vi "Multiple QCM VI.vi"() -> ()   [LabVIEW 2014]
uses:
  <vilib>/Utility/error.llb/DialogType.ctl
  <vilib>/Instr/_visa.llb/VISA Configure Serial Port (Instr).vi
  <vilib>/DAQmx/create/channels.llb/DAQmx Create Channel (DO-Digital Output).vi
  <vilib>/DAQmx/write.llb/DAQmx Write (Digital 1D Bool 1Chan 1Samp).vi
  <vilib>/Utility/file.llb/Write To Spreadsheet File (string).vi
  <vilib>/Utility/file.llb/Write To Spreadsheet File (DBL).vi
panel:
  out "x-y 3":dbl
  out "x-y 2":dbl
  out "Numeric":i32
  out "s? t:f 3":dbl
  out "Waveform Chart 8":dbl[](graph) caption="Waveform Chart"
  out "Frequency 3":dbl
  out "X":dbl
  out "x-y":dbl
  out "s? t:f 2":dbl
  out "Waveform Chart 7":dbl[](graph) caption="Waveform Chart"
  out "Y":dbl
  out "Waveform Chart 6":dbl[](graph) caption="Waveform Chart"
  out "y":dbl
  in  "stop":bool
  out "Frequency 2":dbl
  out "Frequency":dbl
  out "Waveform Chart 2":dbl[](graph) caption="Waveform Chart"
  out "Temperature":dbl
  out "Current Channel\nEnabled":dbl
  out "read buffer":string
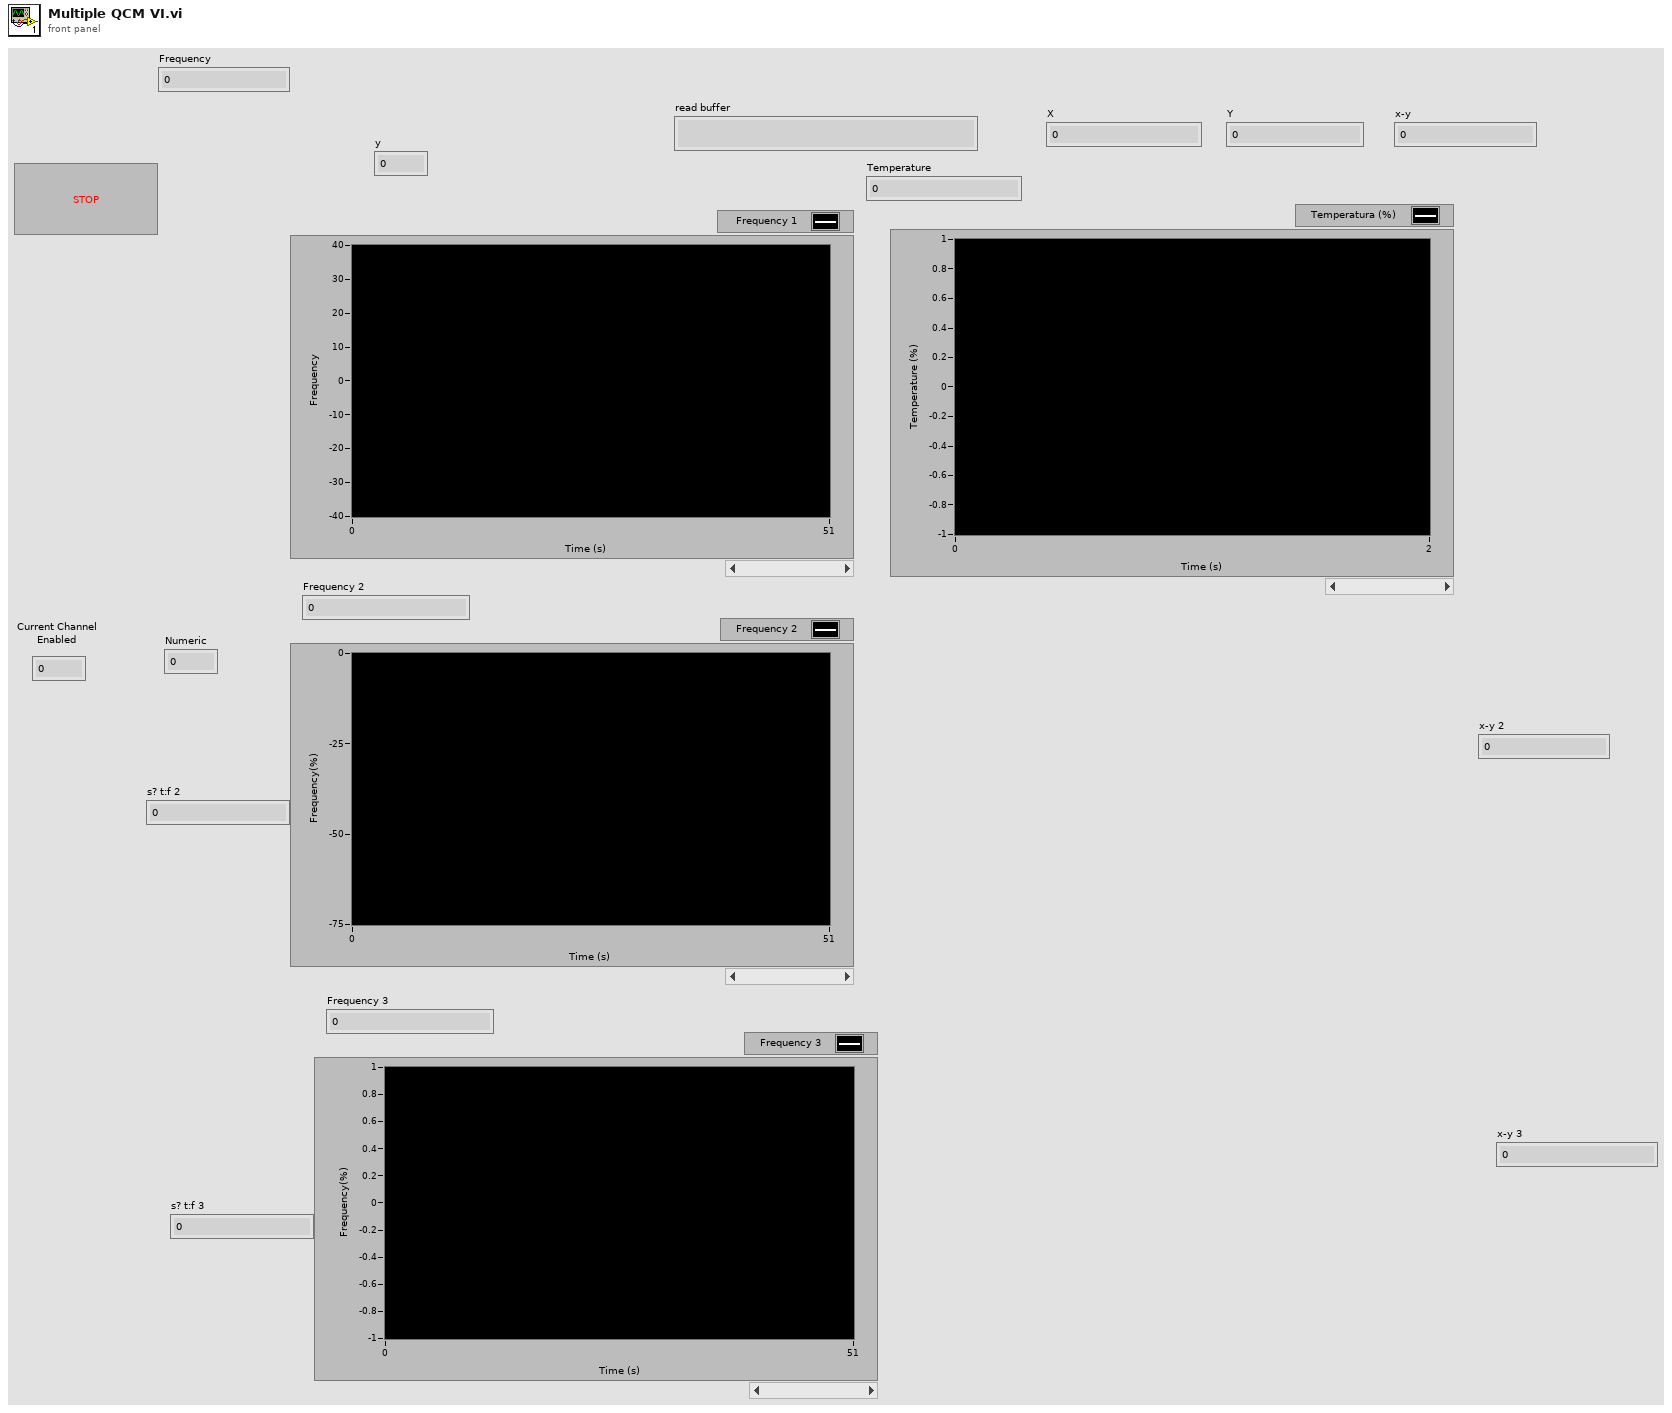
[diagram p1: front panel]
types:
  T1 = typedef "DialogType.ctl" = u16
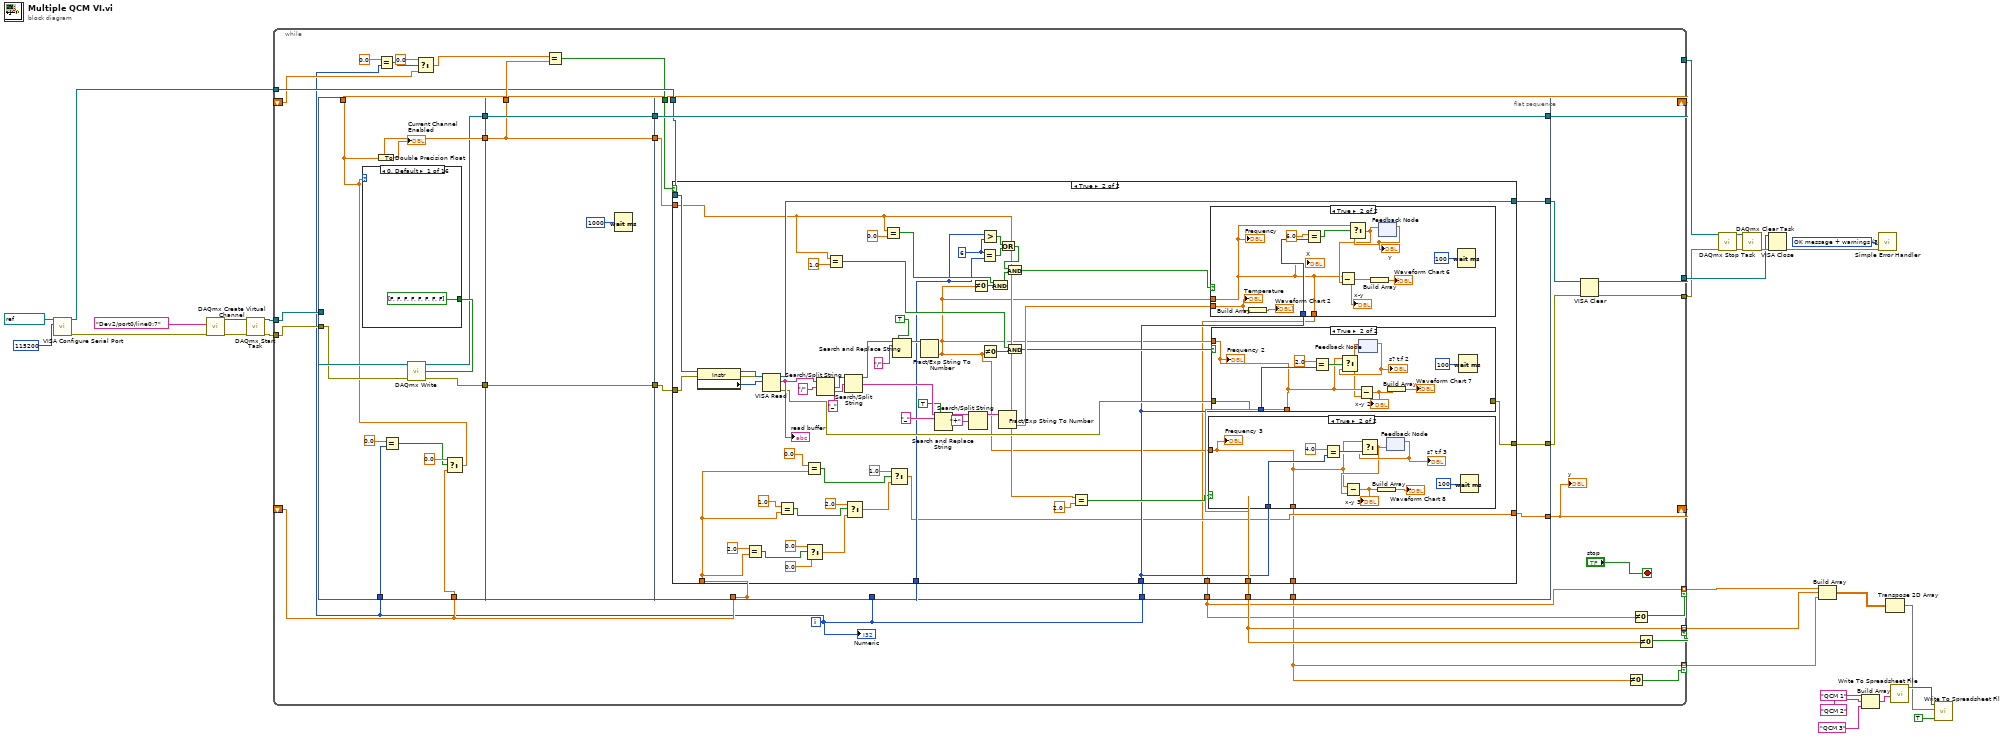
[diagram p0: block diagram]
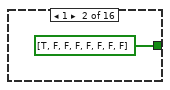
[diagram p2: hidden frame]
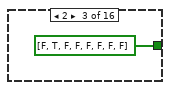
[diagram p3: hidden frame]
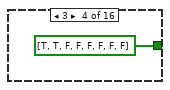
[diagram p4: hidden frame]
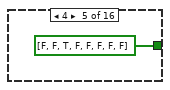
[diagram p5: hidden frame]
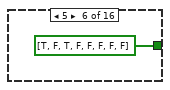
[diagram p6: hidden frame]
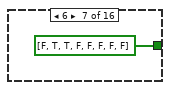
[diagram p7: hidden frame]
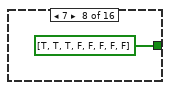
[diagram p8: hidden frame]
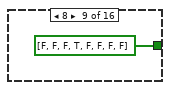
[diagram p9: hidden frame]
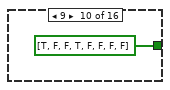
[diagram p10: hidden frame]
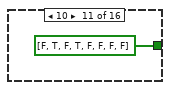
[diagram p11: hidden frame]
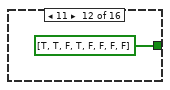
[diagram p12: hidden frame]
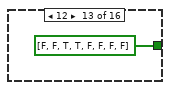
[diagram p13: hidden frame]
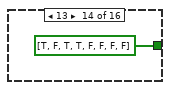
[diagram p14: hidden frame]
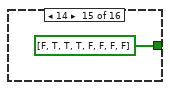
[diagram p15: hidden frame]
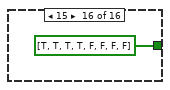
[diagram p16: hidden frame]
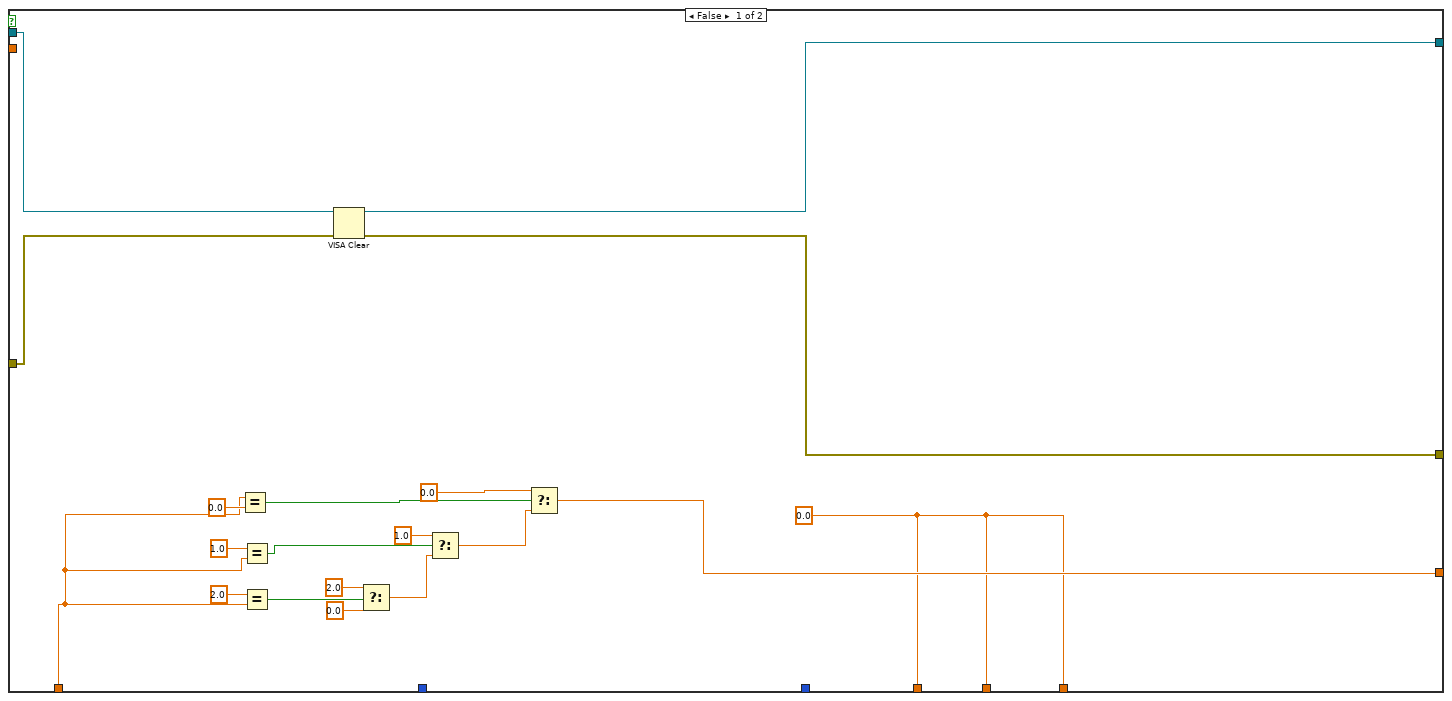
[diagram p17: hidden frame]
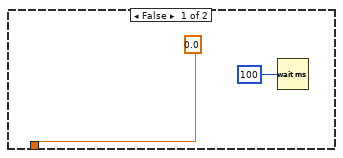
[diagram p18: hidden frame]
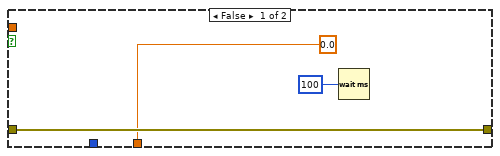
[diagram p19: hidden frame]
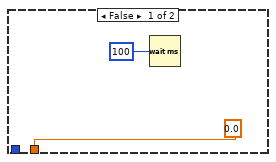
[diagram p20: hidden frame]
diagram:
  w25 = T1 3 items=["no dialog", "OK message", "continue or stop message", "OK message + warnings", "continue/stop + warnings"] ("type of dialog (OK msg:1)")
  n1 = call-poly "VISA Configure Serial Port"("VISA resource name"=refnum<visa-resource-name> "COM12", "baud rate (9600)"=u32 115200) -> ("VISA resource name out"=w28:refnum<visa-resource-name>, "error out"=w19:errorcluster)  [unwired: 12 in]
  n2 = call-poly <vilib>:"DAQmx Create Virtual Channel.vi"("lines"=tag "Dev2/port0/line0:7" ("Line(s)"), "error in"=w19) -> ("task out"=w22:refnum<k21>, "error out"=w21:errorcluster)  [unwired: 12 in]
  n3 = call <vilib>:"DAQmx Start Task.vi"("task/channels in"=w22, "error in"=w21) -> ("task out"=w18:refnum<k21>, "error out"=w17:errorcluster)  [unwired: 12 in]
  n4 = while {
    tunnel: w28 -> [w47]
    tunnel: w18 -> [w58]
    tunnel: w17 -> [w59]
    shift-right: [w43] -> _
    shift-left: _ -> [w36]
    tunnel: [w52] -> w3
    tunnel: [w53] -> w14
    tunnel: [w57] -> w2
    shift-right: [w33] -> _
    shift-left: _ -> [w40]
    tunnel: [w31] -> w6 mode=indexing if=w41
    tunnel: [w32] -> w5 mode=indexing if=w42
    tunnel: [w29] -> w1 mode=indexing if=w30
    i -> [w34]
    stop <- "stop" stop-if-true
    n5 = flat-sequence {
      tunnel: w59 -> [w68]
      tunnel: w58 -> [w71]
      tunnel: [w70] -> w56
      tunnel: [w62] -> w55
      tunnel: [w69] -> w54
      tunnel: w40 -> [w64]
      tunnel: [w61] -> w43
      tunnel: w34 -> [w66]
      tunnel: w56 -> [w90]
      tunnel: w55 -> [w92]
      tunnel: w54 -> [w91]
      tunnel: [w90] -> w51
      tunnel: [w90] -> w50
      tunnel: [w92] -> w49
      tunnel: [w91] -> w48
      tunnel: w50 -> [w103]
      tunnel: w49 -> [w102]
      tunnel: w48 -> [w106]
      tunnel: w47 -> [w105]
      tunnel: w46 -> [w104]
      tunnel: [w97] -> _
      tunnel: [w99] -> w31
      tunnel: [w95] -> w32
      tunnel: w34 -> [w98]
      tunnel: w40 -> [w97]
      tunnel: w34 -> [w96]
      tunnel: [w106] -> w57
      tunnel: [w94] -> w44
      tunnel: [w101] -> w45
      tunnel: [w100] -> w33
      tunnel: [w93] -> w29
      frame #0 {
        n6 = Equal?(x=0.0, y=w66) -> (x = y?=w63:bool)
        n7 = Select(t=0.0, s=w63, f=w64) -> (s? t:f=w61:dbl)
        n8 = case shown="0, Default" w61 {
          tunnel: [bool[] [FALSE, FALSE, FALSE, FALSE, FALSE, FALSE, FALSE, FALSE] ("Output Array") bool[] [TRUE, FALSE, FALSE, FALSE, FALSE, FALSE, FALSE, FALSE] ("Output Array") bool[] [FALSE, TRUE, FALSE, FALSE, FALSE, FALSE, FALSE, FALSE] ("Output Array") bool[] [TRUE, TRUE, FALSE, FALSE, FALSE, FALSE, FALSE, FALSE] ("Output Array") bool[] [FALSE, FALSE, TRUE, FALSE, FALSE, FALSE, FALSE, FALSE] ("Output Array") bool[] [TRUE, FALSE, TRUE, FALSE, FALSE, FALSE, FALSE, FALSE] ("Output Array") bool[] [FALSE, TRUE, TRUE, FALSE, FALSE, FALSE, FALSE, FALSE] ("Output Array") bool[] [TRUE, TRUE, TRUE, FALSE, FALSE, FALSE, FALSE, FALSE] ("Output Array") bool[] [FALSE, FALSE, FALSE, TRUE, FALSE, FALSE, FALSE, FALSE] ("Output Array") bool[] [TRUE, FALSE, FALSE, TRUE, FALSE, FALSE, FALSE, FALSE] ("Output Array") bool[] [FALSE, TRUE, FALSE, TRUE, FALSE, FALSE, FALSE, FALSE] ("Output Array") bool[] [TRUE, TRUE, FALSE, TRUE, FALSE, FALSE, FALSE, FALSE] ("Output Array") bool[] [FALSE, FALSE, TRUE, TRUE, FALSE, FALSE, FALSE, FALSE] ("Output Array") bool[] [TRUE, FALSE, TRUE, TRUE, FALSE, FALSE, FALSE, FALSE] ("Output Array") bool[] [FALSE, TRUE, TRUE, TRUE, FALSE, FALSE, FALSE, FALSE] ("Output Array") bool[] [TRUE, TRUE, TRUE, TRUE, FALSE, FALSE, FALSE, FALSE] ("Output Array")] -> w72
          frame 0, Default {
          }
          frame 1 {
          }
          frame 2 {
          }
          frame 3 {
          }
          frame 4 {
          }
          frame 5 {
          }
          frame 6 {
          }
          frame 7 {
          }
          frame 8 {
          }
          frame 9 {
          }
          frame 10 {
          }
          frame 11 {
          }
          frame 12 {
          }
          frame 13 {
          }
          frame 14 {
          }
          frame 15 {
          }
        }
        n9 = To Double Precision Float(number=w61) -> (double precision float=w70:dbl)
        "Current Channel\nEnabled" <- w70
        n10 = call-poly <vilib>:"DAQmx Write.vi"("task/channels in"=w71, "data"=w72, "error in"=w68) -> ("task out"=w69:refnum<k21>, "error out"=w62:errorcluster)  [unwired: 10 in, 1 out]
      }
      frame #1 {
        n11 = Wait (ms)(milliseconds to wait=u32 1000) -> ()  [unwired: 1 out]
      }
      frame #2 {
        n12 = case shown="True" w104 {
          tunnel: w105 -> [w123 w166]
          tunnel: w103 -> [_ w145]
          tunnel: w102 -> [w125 w165]
          tunnel: [w124 w155] -> w101
          tunnel: [w122 w164] -> w94
          tunnel: w97 -> [w113 w131]
          tunnel: [w118 w141] -> w100
          tunnel: [w107 w127] -> w99
          tunnel: [w107 w154] -> w95
          tunnel: w98 -> [_ w143]
          tunnel: w96 -> [_ w147]
          tunnel: [w107 w126] -> w93
          frame False {
            w107 = 0.0
            n13 = Equal?(x=w113, y=0.0) -> (x = y?=w120:bool)
            n14 = Equal?(x=1.0, y=w113) -> (x = y?=w116:bool)
            n15 = Equal?(x=2.0, y=w113) -> (x = y?=w111:bool)
            n16 = VISA Clear(VISA resource name=w123, error in (no error)=w125) -> (VISA resource name out=w122:refnum<visa-resource-name>, error out=w124:errorcluster)
            n17 = Select(t=2.0, s=w111, f=0.0) -> (s? t:f=w109:dbl)
            n18 = Select(t=1.0, s=w116, f=w109) -> (s? t:f=w114:dbl)
            n19 = Select(t=0.0, s=w120, f=w114) -> (s? t:f=w118:dbl)
          }
          frame True {
            w148 = 6 ("x")
            n20 = property class="Instr"(reference=w166, error in=w165) -> (reference out=w169:refnum<visa-resource-name>, error out=w167:errorcluster, "Serial Settings:Number of Bytes at Serial Port"=w168:u32)
            n21 = Equal?(x=2.0, y=w131) -> (x = y?=w137:bool)
            n22 = VISA Read(VISA resource name=w169, byte count=w168, error in (no error)=w167) -> (VISA resource name out=w164:refnum<visa-resource-name>, read buffer=w160:string, error out=w156:errorcluster)  [unwired: 1 out]
            "read buffer" <- w160
            n23 = Equal?(x=1.0, y=w131) -> (x = y?=w136:bool)
            n24 = Equal?(x=0.0, y=w131) -> (x = y?=w135:bool)
            n25 = Select(t=0.0, s=w137, f=0.0) -> (s? t:f=w129:dbl)
            n26 = Search/Split String(string=w160, search string/char (-)="/") -> (match + rest of string=w177:string)  [unwired: 1 in, 2 out]
            n27 = Equal?(x=w145, y=1.0) -> (x = y?=w161:bool)
            n28 = Search/Split String(string=w177, search string/char (-)="_") -> (substring before match=w176:string, match + rest of string=w173:string)  [unwired: 1 in, 1 out]
            n29 = Select(t=2.0, s=w136, f=w129) -> (s? t:f=w133:dbl)
            n30 = Equal?(x=w145, y=0.0) -> (x = y?=w162:bool)
            n31 = Select(t=1.0, s=w135, f=w133) -> (s? t:f=w141:dbl)
            n32 = Search and Replace String(replace all?=TRUE ("replace all? (F)"), input string=w176, search string="/" ("replace string (\"\")")) -> (result string=w170:string)  [unwired: 5 in, 3 out]
            n33 = Fract/Exp String To Number(string=w170) -> (number=w142:dbl)  [unwired: 3 in, 1 out]
            n34 = Search and Replace String(replace all?=TRUE ("replace all? (F)"), input string=w173, search string="_") -> (result string=w158:string)  [unwired: 5 in, 3 out]
            n35 = Search/Split String(string=w158, search string/char (-)="+") -> (substring before match=w159:string)  [unwired: 1 in, 2 out]
            n36 = Not Equal To 0?(x=w142) -> (x != 0?=w180:bool)
            n37 = Equal?(x=w148, y=w147) -> (x = y?=w150:bool)
            n38 = Greater?(x=w147, y=w148) -> (0:w149:bool)
            n39 = Not Equal To 0?(x=w142) -> (x != 0?=w182:bool)
            n40 = And(x=w162, y=w180) -> (x .and. y?=w152:bool)
            n41 = Fract/Exp String To Number(string=w159) -> (number=w184:dbl)  [unwired: 3 in, 1 out]
            n42 = Or(x=w149, y=w150) -> (x .or. y?=w151:bool)
            n43 = And(x=w151, y=w152) -> (x .and. y?=w153:bool)
            n44 = And(x=w161, y=w182) -> (x .and. y?=w183:bool)
            n45 = Equal?(x=w145, y=2.0) -> (x = y?=w144:bool)
            n46 = case shown="True" w144 {
              tunnel: [0.0 w187] -> w126
              tunnel: w143 -> [_ w190]
              tunnel: w142 -> [_ w187]
              frame False {
                n47 = Wait (ms)(milliseconds to wait=u32 100) -> ()  [unwired: 1 out]
              }
              frame True {
                n48 = Equal?(x=4.0, y=w190) -> (x = y?=w192:bool)
                n49 = feedback #1() -> (w191:dbl)  [unwired: 1 in]
                "s? t:f 3" <- w191
                n50 = Select(t=w187, s=w192, f=w191) -> (s? t:f=w188:dbl)
                n51 = Subtract(x=w187, y=w188) -> (x-y=w193:dbl)
                "x-y 3" <- w193
                n52 = Build Array(w193) -> (→"Waveform Chart 8":dbl[])
                n53 = feedback-in #1(w188) -> ()
                n54 = Wait (ms)(milliseconds to wait=u32 100) -> ()  [unwired: 1 out]
                "Frequency 3" <- w187
              }
            }
            n55 = case shown="True" w153 {
              tunnel: w142 -> [_ w211]
              tunnel: w184 -> [_ w220]
              tunnel: [0.0 w211] -> w127
              tunnel: w143 -> [_ w218]
              frame False {
                n56 = Wait (ms)(milliseconds to wait=u32 100) -> ()  [unwired: 1 out]
              }
              frame True {
                n57 = Build Array(w220) -> (→"Waveform Chart 2":dbl[])
                n58 = Equal?(x=6.0, y=w218) -> (x = y?=w215:bool)
                n59 = feedback #2() -> (w214:dbl)  [unwired: 1 in]
                "Y" <- w214
                n60 = Select(t=w211, s=w215, f=w214) -> (s? t:f=w213:dbl)
                n61 = Subtract(x=w211, y=w213) -> (x-y=w216:dbl)
                "x-y" <- w216
                n62 = Build Array(w216) -> (→"Waveform Chart 6":dbl[])
                n63 = feedback-in #2(w213) -> ()
                n64 = Wait (ms)(milliseconds to wait=u32 100) -> ()  [unwired: 1 out]
                "Temperature" <- w220
                "Frequency" <- w211
                "X" <- w211
              }
            }
            n65 = case shown="True" w183 {
              tunnel: w142 -> [_ w201]
              tunnel: w156 -> [w198 w208]
              tunnel: [w198 w208] -> w155
              tunnel: [0.0 w201] -> w154
              tunnel: w143 -> [_ w203]
              frame False {
                n66 = Wait (ms)(milliseconds to wait=u32 100) -> ()  [unwired: 1 out]
              }
              frame True {
                n67 = Equal?(x=2.0, y=w203) -> (x = y?=w204:bool)
                n68 = feedback #3() -> (w202:dbl)  [unwired: 1 in]
                "s? t:f 2" <- w202
                n69 = Select(t=w201, s=w204, f=w202) -> (s? t:f=w200:dbl)
                n70 = Subtract(x=w201, y=w200) -> (x-y=w205:dbl)
                "x-y 2" <- w205
                n71 = feedback-in #3(w200) -> ()
                n72 = Build Array(w205) -> (→"Waveform Chart 7":dbl[])
                n73 = Wait (ms)(milliseconds to wait=u32 100) -> ()  [unwired: 1 out]
                "Frequency 2" <- w201
              }
            }
          }
        }
      }
    }
    n74 = Equal?(x=0.0, y=w34) -> (x = y?=w38:bool)
    n75 = Select(t=0.0, s=w38, f=w36) -> (s? t:f=w35:dbl)
    n76 = Equal?(x=w35, y=w51) -> (x = y?=w46:bool)
    n77 = VISA Clear(VISA resource name=w44, error in (no error)=w45) -> (VISA resource name out=w53:refnum<visa-resource-name>, error out=w52:errorcluster)
    n78 = Not Equal To 0?(x=w29) -> (x != 0?=w30:bool)
    n79 = Not Equal To 0?(x=w31) -> (x != 0?=w41:bool)
    n80 = Not Equal To 0?(x=w32) -> (x != 0?=w42:bool)
    "Numeric" <- w34
    "y" <- w33
  }
  n81 = call <vilib>:"DAQmx Stop Task.vi"("task/channels in"=w2, "error in"=w3) -> ("task out"=w23:refnum<k21>, "error out"=w24:errorcluster)  [unwired: 12 in]
  n82 = call <vilib>:"DAQmx Clear Task.vi"("task in"=w23, "error in"=w24) -> ("error out"=w16:errorcluster)  [unwired: 13 in]
  n83 = VISA Close(VISA resource name=w14, error in (no error)=w16) -> (error out=w15:errorcluster)
  n84 = Build Array(w6, w5, w1) -> (w8:dbl[][])
  n85 = Build Array("QCM 1", "QCM 2", "QCM 3" ("element")) -> (w11:string[])
  n86 = call <vilib>:"Simple Error Handler.vi"("type of dialog (OK msg:1)"=w25, "error in (no error)"=w15) -> ()  [unwired: 3 in, 5 out]
  n87 = Transpose 2D Array(2D array=w8) -> (transposed array=w7:dbl[][])
  n88 = call-poly <vilib>:"Write To Spreadsheet File.vi"("1D data"=w11) -> ("new file path (Not A Path if cancelled)"=w12:path)  [unwired: 7 in]
  n89 = call-poly <vilib>:"Write To Spreadsheet File.vi"("append to file? (new file:F)"=TRUE, "2D data"=w7, "file path (dialog if empty)"=w12) -> ()  [unwired: 5 in, 1 out]
